vi "Command Detect Time (SubVI).vi"(10 "Read String":string, 11 "Boolean in":bool) -> (2 "String":string, 3 "Boolean out":bool)   [LabVIEW 2014]
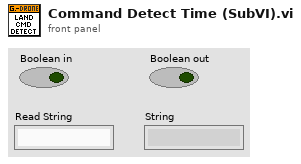
[diagram p1: front panel]
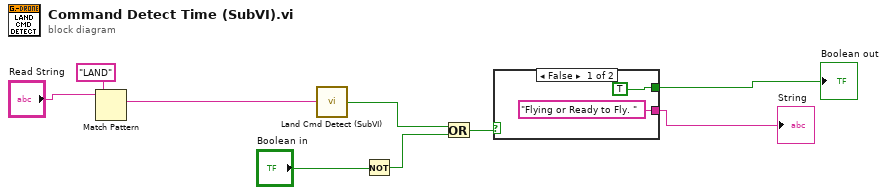
[diagram p0: block diagram]
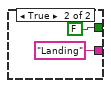
[diagram p2: hidden frame]
diagram:
  n1 = Match Pattern(string="Read String", regular expression="LAND") -> (match substring=w7:string)  [unwired: 1 in, 3 out]
  n2 = call "Land Cmd Detect (SubVI).vi"("Read String"=w7) -> ("Land Command"=w4:bool)
  n3 = Not(x="Boolean in") -> (.not. x?=w2:bool)
  n4 = Or(x=w4, y=w2) -> (x .or. y?=w1:bool)
  n5 = case shown="False" w1 {
    tunnel: [TRUE FALSE] -> w5
    tunnel: ["Flying or Ready to Fly. " "Landing"] -> w9
    frame False {
    }
    frame True {
    }
  }
  "String" <- w9
  "Boolean out" <- w5
